vi "MyrioProject.vi"() -> ()   [LabVIEW 2018]
doc: "The myRIO Project template acquires acceleration data from the onboard accelerometer and displays the changes of acceleration values in a waveform chart."
uses:
  <vilib>/Platform/TimedLoop/XDataNode/timing_clust.ctl
  <vilib>/Platform/TimedLoop/XDataNode/nitl_modes.ctl
  <vilib>/Platform/TimedLoop/XDataNode/wakeup.ctl
  <vilib>/myRIO/Common/Instrument Driver Framework/myRIO v1.0/Encoder/typedefs/Encoder Signal Mode.ctl
  <vilib>/myRIO/Instrument Drivers/Onboard IO/PWM/typedefs/PWM Reference.ctl
  <vilib>/myRIO/Common/Instrument Driver Framework/Utilities/typedefs/myRIO Generic Hardware Reference.ctl
  <vilib>/myRIO/Common/Instrument Driver Framework/Utilities/typedefs/Hardware Version Enum.ctl
  <vilib>/myRIO/Common/Instrument Driver Framework/Utilities/typedefs/myRIO v1.0 Reference.ctl
  <vilib>/myRIO/Common/Instrument Driver Framework/Utilities/typedefs/Generic FPGA Reference.ctl
  <vilib>/myRIO/Common/Instrument Driver Framework/myRIO v1.0/PWM/typedefs/PWM Channels Enum.ctl
  <vilib>/myRIO/Instrument Drivers/Onboard IO/PWM/typedefs/PWM Configuration.ctl
  <vilib>/userdefined/High Color/nirio_resource_hc.ctl
  <vilib>/myRIO/Common/Instrument Driver Framework/myRIO v1.0/Encoder/typedefs/Encoder Configuration v1.0.ctl
  <vilib>/myRIO/Instrument Drivers/Onboard IO/Encoder/typedefs/Encoder Reference.ctl
  <vilib>/myRIO/Common/Instrument Driver Framework/myRIO v1.0/Encoder/typedefs/Encoder Channels Enum.ctl
  <vilib>/myRIO/Instrument Drivers/Onboard IO/DIO/typedefs/DIO Reference.ctl
  <vilib>/myRIO/Common/Instrument Driver Framework/myRIO v1.0/DIO/typedefs/DIO Channels List.ctl
  <vilib>/myRIO/Common/Instrument Driver Framework/myRIO v1.0/DIO/typedefs/DIO Channels Enum.ctl
  <vilib>/myRIO/Instrument Drivers/Onboard IO/AI/typedefs/AI Reference.ctl
  <vilib>/myRIO/Common/Instrument Driver Framework/myRIO v1.0/AI/typedefs/AI Channels List.ctl
  <vilib>/myRIO/Common/Instrument Driver Framework/myRIO v1.0/AI/typedefs/AI Channels Enum.ctl
  <vilib>/myRIO/Common/Instrument Driver Framework/Utilities/typedefs/Analog Scaling Constants List.ctl
  <vilib>/myRIO/Common/Instrument Driver Framework/Utilities/typedefs/Analog Scaling Constants.ctl
  <vilib>/myRIO/Common/Instrument Driver Framework/myRIO v1.0/PWM/vis/myRIO v1.1 Open PWM.vi
  <vilib>/myRIO/Common/Instrument Driver Framework/myRIO v1.0/Encoder/vis/myRIO v1.1 Open Encoder.vi
  <vilib>/myRIO/Common/Instrument Driver Framework/Utilities/vis/Is FPGA Ref Available.vi
  <vilib>/myRIO/Common/Instrument Driver Framework/myRIO v1.0/AI/vis/myRIO v1.1 Open AI.vi
  <vilib>/myRIO/Common/Instrument Driver Framework/myRIO v1.0/DIO/vis/myRIO v1.1 Open DIO.vi
  <vilib>/myRIO/Instrument Drivers/Onboard IO/PWM/vis/Set Duty Cycle and Frequency.vi
  <vilib>/myRIO/Instrument Drivers/Onboard IO/DIO/vis/Write.vi
  <vilib>/myRIO/Common/Instrument Driver Framework/Utilities/vis/Validate Channels.vi
  <vilib>/myRIO/Common/Instrument Driver Framework/myRIO v1.0/PWM/vis/myRIO v1.0 Reserve PWM.vi
  <vilib>/myRIO/Common/Instrument Driver Framework/myRIO v1.0/Encoder/vis/myRIO v1.0 Reserve Encoder.vi
  <vilib>/myRIO/Common/Instrument Driver Framework/myRIO v1.0/AI/vis/myRIO v1.0 Reserve AI.vi
  <vilib>/myRIO/Common/Instrument Driver Framework/myRIO v1.0/DIO/vis/myRIO v1.0 Reserve DIO.vi
  <vilib>/myRIO/Common/Instrument Driver Framework/myRIO v1.0/Encoder/vis/myRIO v1.0 Close Encoder.vi
  <vilib>/myRIO/Common/Instrument Driver Framework/myRIO v1.0/PWM/vis/myRIO v1.0 Close PWM.vi
  <vilib>/myRIO/Common/Instrument Driver Framework/myRIO v1.0/PWM/vis/myRIO v1.0 Build MUX Configuration PWM.vi
  <vilib>/myRIO/Common/Instrument Driver Framework/myRIO v1.0/Resource Manager/vis/myRIO v1.0 Reserve Channel List.vi
  <vilib>/myRIO/Common/Instrument Driver Framework/myRIO v1.0/Encoder/vis/myRIO v1.0 Build MUX Configuration Encoder.vi
  <vilib>/myRIO/Common/Instrument Driver Framework/myRIO v1.0/AI/vis/myRIO v1.0 Build MUX Configuration AI.vi
  <vilib>/myRIO/Common/Instrument Driver Framework/myRIO v1.0/DIO/vis/myRIO v1.0 Build MUX Configuration DIO.vi
  <vilib>/myRIO/Common/Instrument Driver Framework/myRIO v1.0/Encoder/vis/myRIO v1.0 Unreserve Encoder.vi
  <vilib>/myRIO/Common/Instrument Driver Framework/myRIO v1.0/PWM/vis/myRIO v1.0 Unreserve PWM.vi
  <vilib>/myRIO/Common/Instrument Driver Framework/myRIO v1.0/Resource Manager/vis/myRIO v1.0 Create Configuration List.vi
  <vilib>/myRIO/Common/Instrument Driver Framework/myRIO v1.0/Resource Manager/vis/myRIO v1.0 Reserve Channel.vi
  <vilib>/myRIO/Common/Instrument Driver Framework/myRIO v1.0/Resource Manager/vis/myRIO v1.0 Unreserve Channel.vi
  <vilib>/myRIO/Common/Instrument Driver Framework/myRIO v1.0/Resource Manager/vis/myRIO v1.0 Unreserve Channel List.vi
  <vilib>/myRIO/Common/Instrument Driver Framework/myRIO v1.0/Resource Manager/vis/myRIO v1.0 Build Mutex Name.vi
  <vilib>/Utility/VariantDataType/GetNumericInfo.vi
  <vilib>/Utility/error.llb/Error Cluster From Error Code.vi
  <vilib>/myRIO/Common/Instrument Driver Framework/myRIO v1.0/myRIO v1.1 Open.vi
  <vilib>/myRIO/Common/Instrument Driver Framework/Utilities/vis/IO Manager.vi
  <vilib>/myRIO/Common/Instrument Driver Framework/Utilities/vis/Configuration Manager.vi
  <vilib>/myRIO/Common/Instrument Driver Framework/myRIO v1.0/Resource Manager/vis/myRIO v1.0 Configure IO.vi
  <vilib>/myRIO/Common/Instrument Driver Framework/myRIO v1.0/myRIO v1.0 Close.vi
  <vilib>/myRIO/Common/Instrument Driver Framework/myRIO v1.0/PWM/vis/myRIO v1.0 Write PWM.vi
  <vilib>/myRIO/Common/Instrument Driver Framework/myRIO v1.0/Encoder/vis/myRIO v1.0 Configure Encoder.vi
  <vilib>/myRIO/Common/Instrument Driver Framework/myRIO v1.0/Encoder/vis/myRIO v1.0 Enable Encoder.vi
  <vilib>/myRIO/Common/Instrument Driver Framework/myRIO v1.0/DIO/vis/myRIO v1.0 Read DIO.vi
  <vilib>/myRIO/Common/Instrument Driver Framework/myRIO v1.0/AI/vis/myRIO v1.0 Get Scaling Constants AI.vi
  <vilib>/myRIO/Common/Instrument Driver Framework/myRIO v1.0/AI/vis/myRIO v1.0 Read AI.vi
  <vilib>/myRIO/Common/Instrument Driver Framework/myRIO v1.0/Encoder/vis/myRIO v1.0 Read Encoder.vi
  <vilib>/myRIO/Common/Instrument Driver Framework/myRIO v1.0/DIO/vis/myRIO v1.0 Write DIO.vi
  <vilib>/myRIO/Common/Instrument Driver Framework/myRIO v1.0/Encoder/vis/myRIO v1.0 Shutdown Encoder.vi
  <vilib>/myRIO/Common/Instrument Driver Framework/myRIO v1.0/PWM/vis/myRIO v1.0 Shutdown PWM.vi
  <vilib>/platform/TimedLoop/XDataNode/XDataNode.xnode
  <vilib>/myRIO/Instrument Drivers/Onboard IO/PWM/vis/myRIO PWM Open.xnode
  <vilib>/myRIO/Instrument Drivers/Onboard IO/Encoder/vis/myRIO Encoder Open.xnode
  <vilib>/myRIO/Express VI/Onboard IO/PWM/PWM Express VI.xnode
  <vilib>/myRIO/Express VI/Onboard Devices/Button/Button Express VI.xnode
  <vilib>/myRIO/Instrument Drivers/Onboard IO/DIO/vis/myRIO DIO Open.xnode
  <vilib>/myRIO/Express VI/Onboard IO/AI/AI Express VI.xnode
  <vilib>/myRIO/Instrument Drivers/Onboard IO/AI/vis/myRIO AI Open.xnode
  <vilib>/myRIO/Express VI/Onboard IO/DO/DO Express VI.xnode
  <vilib>/Platform/TimedLoop/XDataNode/XDNodeRunTimeDep.lvlib
  <vilib>/myRIO/Instrument Drivers/Onboard IO/Encoder/Encoder.lvlib
  <vilib>/myRIO/Instrument Drivers/Onboard IO/PWM/PWM.lvlib
  <vilib>/myRIO/Instrument Drivers/Onboard IO/DIO/DIO.lvlib
  <vilib>/myRIO/Instrument Drivers/Onboard IO/AI/AI.lvlib
panel:
  in  "MANUAL 2":bool
  in  "Stop Button":bool
  in  "Start":bool
  out "element":dbl
  out "element 2":dbl
  out "subarray 2":dbl[][](array[numeric])
  out "subarray":dbl[][](array[numeric])
  out "vectores":dbl[][][](array[numeric])
  in  "saturacion":dbl
  in  "Duty Cycle 2":dbl(slide)=0.5 scale=0.05..0.1
  in  "Duty Cycle":dbl(slide)=0.5 scale=0.05..0.1
  in  "Reset Counter 2":bool
  in  "Reset Counter":bool
  out "stallRojo (A/AI3 (Pin 9))":dbl
  out "stallBlanco (A/AI2 (Pin 7))":dbl
  out "sensor2 (A/AI1 (Pin 5))":dbl
  out "A/AI0 (Pin 3)":dbl
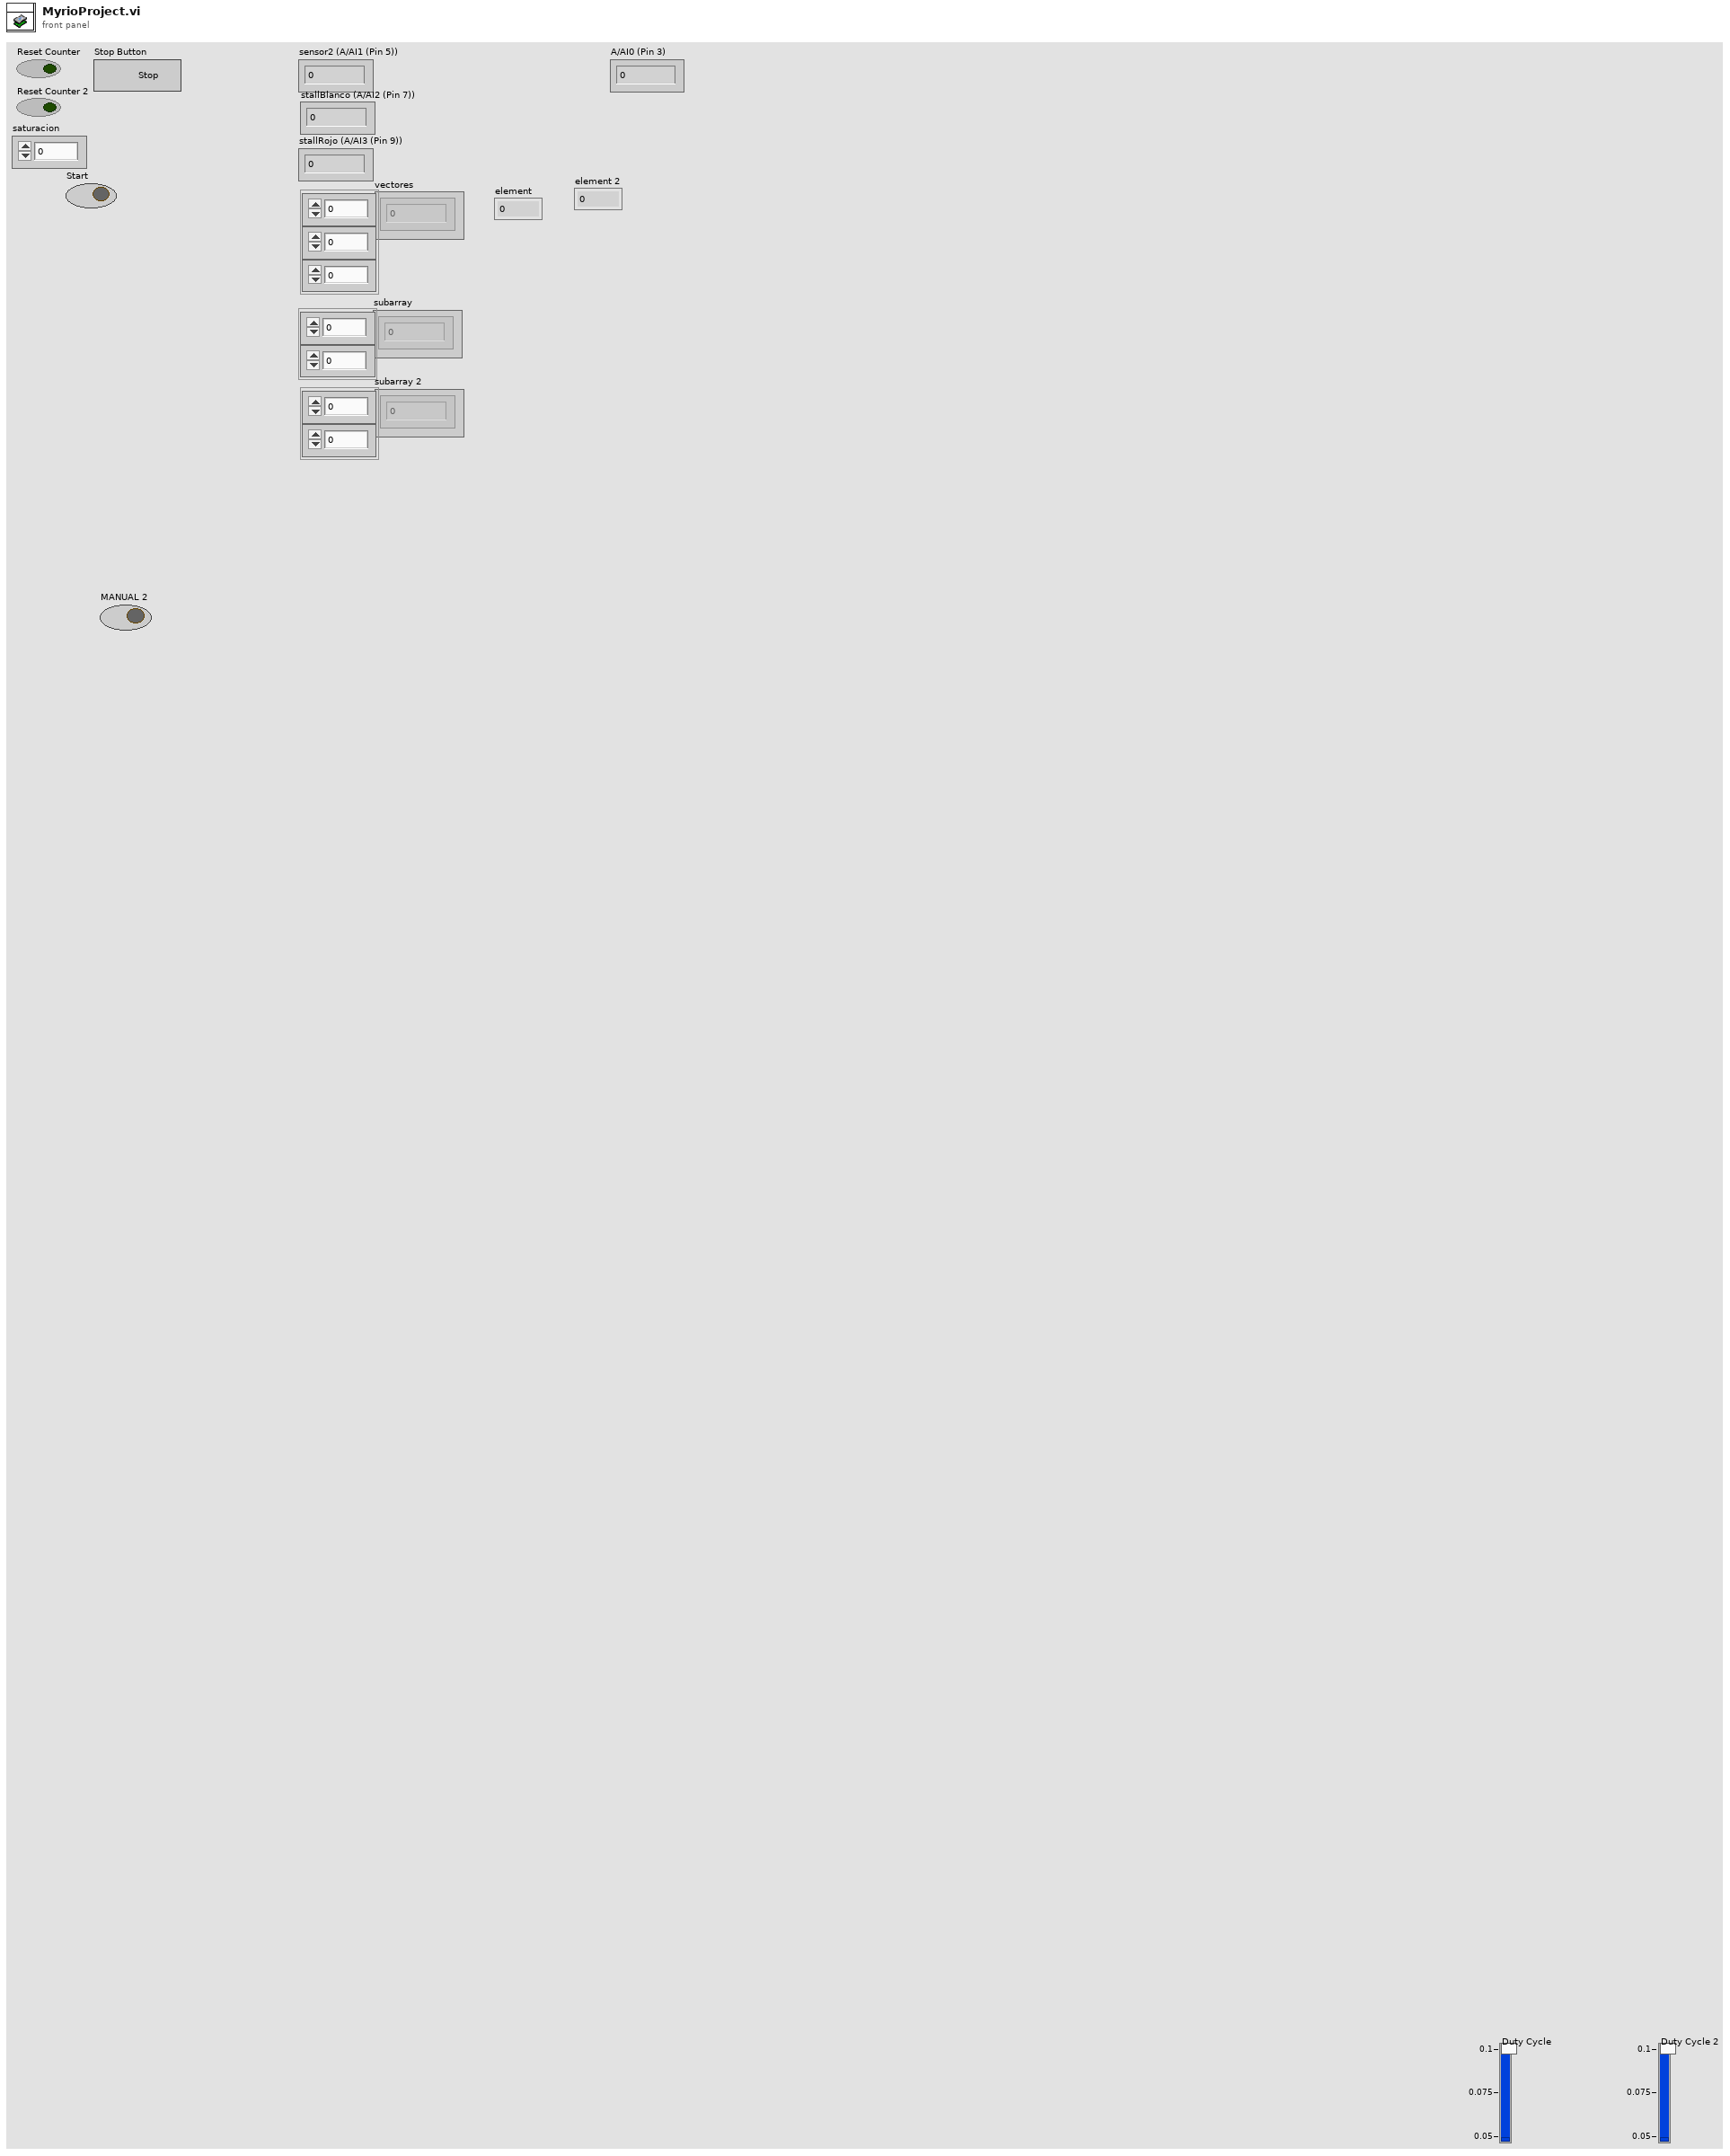
[diagram p1: front panel]
types:
  T1 = typedef "Encoder Signal Mode.ctl" = enum16{"Quadrature phase signal", "Step and direction signal"}
  T2 = typedef "PWM.lvlib/PWM Reference.ctl" = cluster{"myRIO Reference":T3, "PWM Channels Enum":T7, "PWM Configuration":T8}
  T3 = typedef "myRIO Generic Hardware Reference.ctl" = cluster{"myRIO Model":T4, "myRIO Hardware Reference":T5}
  T4 = typedef "Hardware Version Enum.ctl" = enum16{"Unknown", "myRIO-1900", "myRIO-1950", "roboRIO", "NI ELVIS RIO CM", "ELVIS III"}
  T5 = typedef "myRIO v1.0 Reference.ctl" = cluster{"Generic FPGA Reference":T6, "Allow multiple opens":bool}
  T6 = typedef "Generic FPGA Reference.ctl" = refnum<k20>
  T7 = typedef "PWM Channels Enum.ctl" = enum16{"Not Connected", "C/PWM0", "C/PWM1", "A/PWM0", "A/PWM1", "A/PWM2", "A/PWM3", "A/PWM4", "A/PWM5", "A/PWM6", "A/PWM7", "A/PWM8", "A/PWM9", "A/PWM10", "A/PWM11", "A/PWM12", "A/PWM13", "A/PWM14", "A/PWM15", "A/PWM16", "A/PWM17", "A/PWM18", "A/PWM19", "B/PWM0", "B/PWM1", "B/PWM2", "B/PWM3", "B/PWM4", "B/PWM5", "B/PWM6", "B/PWM7", "B/PWM8", "B/PWM9", "B/PWM10", "B/PWM11", "B/PWM12", "B/PWM13", "B/PWM14", "B/PWM15", "B/PWM16", "B/PWM17", "B/PWM18", "B/PWM19", "PWM/PWM0", "PWM/PWM1", "PWM/PWM2", "PWM/PWM3", "PWM/PWM4", "PWM/PWM5", "PWM/PWM6", "PWM/PWM7", "PWM/PWM8", "PWM/PWM9"}
  T8 = typedef "PWM.lvlib/PWM Configuration.ctl" = cluster{"Frequency":dbl, "Duty Cycle":dbl}
  T9 = typedef "Encoder.lvlib/Encoder Reference.ctl" = cluster{"myRIO Reference":T3, "Encoder Channels Enum":T10}
  T10 = typedef "Encoder Channels Enum.ctl" = enum16{"Not Connected", "C/ENC0", "C/ENC1", "A/ENC", "A/ENC0", "A/ENC1", "A/ENC2", "A/ENC3", "A/ENC4", "A/ENC5", "A/ENC6", "A/ENC7", "A/ENC8", "A/ENC9", "B/ENC", "B/ENC0", "B/ENC1", "B/ENC2", "B/ENC3", "B/ENC4", "B/ENC5", "B/ENC6", "B/ENC7", "B/ENC8", "B/ENC9", "DIO/ENC0", "DIO/ENC1", "DIO/ENC2", "DIO/ENC3", "DIO/ENC4"}
  T11 = typedef "XDNodeRunTimeDep.lvlib/timing_clust.ctl" = cluster{"Expected End [f-1]":u64, "Actual End [f-1]":u64, "Finished Late? [f-1]":bool, "Expected End [i-1]":u64, "Actual End [i-1]":u64, "Finished Late? [i-1]":bool, "Expected Start [i]":u64, "Actual Start [i]":u64, "Expected Start [f]":u64, "Actual Start [f]":u64, "Source Name":string, "Structure Name":string, "Period":i64, "Deadline":i64, "Offset":i64, "Start":i64, "Priority":i32, "Timeout":i32, "Mode":T12, "Wakeup Reason":T13, "Error":errorcluster, "Source Type":string, "Secondary Source Type":string, "Global End Time":u64, "Global Start Time":u64, "Frame Duration":u64, "Iteration Duration":u64, "Assigned CPU":i32, "I/O Scan Engine Mode":u32}
  T12 = typedef "XDNodeRunTimeDep.lvlib/nitl_modes.ctl" = enum32{"No Change", "Process missed periods, maintain original phase", "Discard missed periods, maintain original phase", "Process missed periods, ignore original phase", "Discard missed periods, ignore original phase"}
  T13 = typedef "XDNodeRunTimeDep.lvlib/wakeup.ctl" = enum32{"Normal", "Aborted", "Asynchronous wakeup", "Timing source error", "Timed loop error", "Timeout"}
  T14 = enum16{"normal", "grande-Sensor", "grande home", "peque-sensor", "peque- home", "peque-reset"}
  T15 = typedef "nirio_resource_hc.ctl" = tag
  T16 = enum16{"normal", "grande-Sensor", "grande home", "peque-sensor", "peque- home"}
  T17 = typedef "AI.lvlib/AI Reference.ctl" = cluster{"myRIO Reference":T3, "AI Channels List":T18, "AI Scaling Constants List":T20}
  T18 = typedef "AI Channels List.ctl" = T19[]
  T19 = typedef "AI Channels Enum.ctl" = enum16{"Not Connected", "AudioIn/Left", "AudioIn/Right", "C/AI0", "C/AI1", "A/AI0", "A/AI1", "A/AI2", "A/AI3", "A/AI4", "A/AI5", "A/AI6", "A/AI7", "B/AI0", "B/AI1", "B/AI2", "B/AI3", "B/AI4", "B/AI5", "B/AI6", "B/AI7", "AI/AI0", "AI/AI1", "AI/AI2", "AI/AI3", "A/AI0 (DIFF)", "A/AI1 (DIFF)", "A/AI2 (DIFF)", "A/AI3 (DIFF)", "B/AI0 (DIFF)", "B/AI1 (DIFF)", "B/AI2 (DIFF)", "B/AI3 (DIFF)"}
  T20 = typedef "Analog Scaling Constants List.ctl" = T21[]
  T21 = typedef "Analog Scaling Constants.ctl" = cluster{"LSB Weight (Volts)":dbl, "Offset (Volts)":dbl, "Signed?":bool}
  T22 = typedef "DIO.lvlib/DIO Reference.ctl" = cluster{"myRIO Reference":T3, "DIO Channels List":T23}
  T23 = typedef "DIO Channels List.ctl" = T24[]
  T24 = typedef "DIO Channels Enum.ctl" = enum16{"Not Connected", "C/DIO0", "C/DIO1", "C/DIO2", "C/DIO3", "C/DIO4", "C/DIO5", "C/DIO6", "C/DIO7", "A/DIO0", "A/DIO1", "A/DIO2", "A/DIO3", "A/DIO4", "A/DIO5", "A/DIO6", "A/DIO7", "A/DIO8", "A/DIO9", "A/DIO10", "A/DIO11", "A/DIO12", "A/DIO13", "A/DIO14", "A/DIO15", "A/DIO16", "A/DIO17", "A/DIO18", "A/DIO19", "B/DIO0", "B/DIO1", "B/DIO2", "B/DIO3", "B/DIO4", "B/DIO5", "B/DIO6", "B/DIO7", "B/DIO8", "B/DIO9", "B/DIO10", "B/DIO11", "B/DIO12", "B/DIO13", "B/DIO14", "B/DIO15", "B/DIO16", "B/DIO17", "B/DIO18", "B/DIO19", "LED0", "LED1", "LED2", "LED3", "Button0", "DIO/DIO0", "DIO/DIO1", "DIO/DIO2", "DIO/DIO3", "DIO/DIO4", "DIO/DIO5", "DIO/DIO6", "DIO/DIO7", "DIO/DIO8", "DIO/DIO9", "SPI/CS0", "SPI/CS1", "SPI/CS2", "SPI/CS3", "LED RADIO (Green)", "LED RADIO (Red)", "LED COMM (Green)", "LED COMM (Red)", "LED MODE (Green)", "LED MODE (Red)"}
  T25 = cluster{"Double":dbl, dbl, "Counter Value":i32, "seconds since 1Jan1904":timestamp, "Double":dbl, dbl, dbl}
  T26 = cluster{"Double":dbl, "dbl Scaled Value":dbl, "Output":dbl, "seconds since 1Jan1904":timestamp, dbl, dbl, dbl}
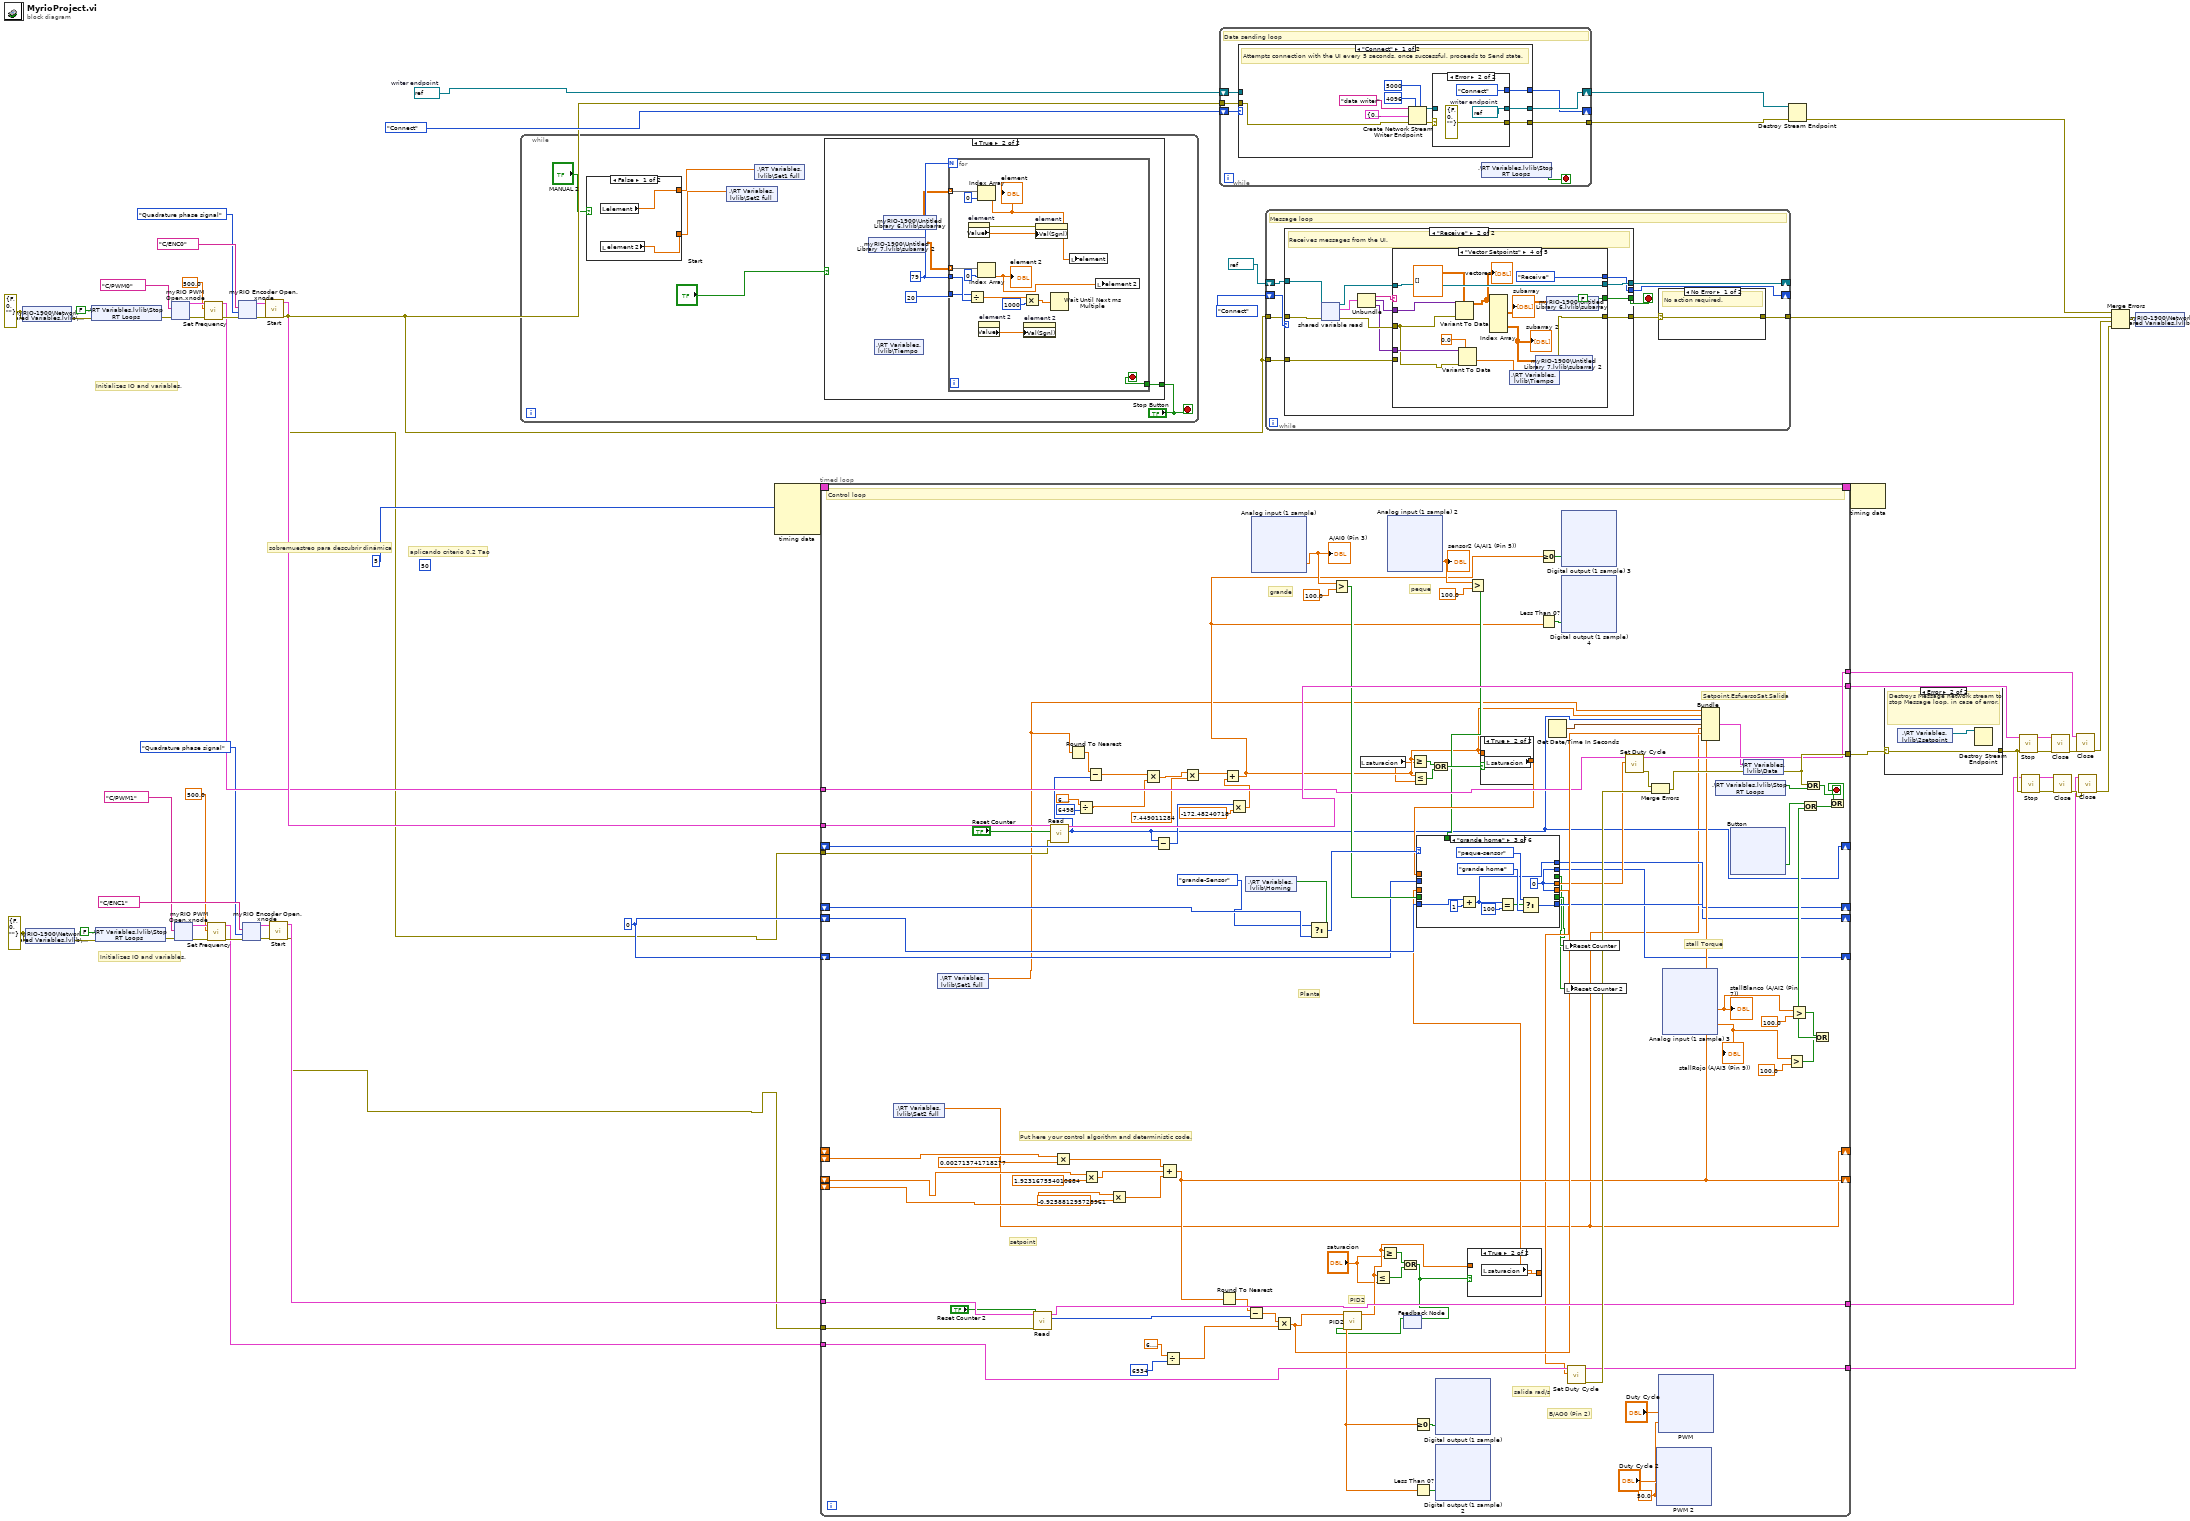
[diagram p0: block diagram]
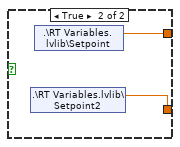
[diagram p2: hidden frame]
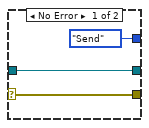
[diagram p5: hidden frame]
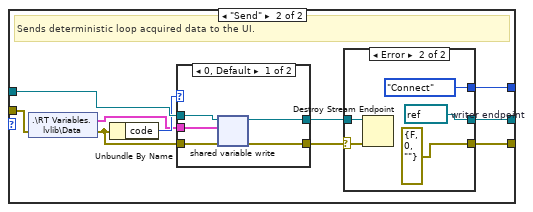
[diagram p6: hidden frame]
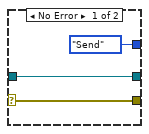
[diagram p7: hidden frame]
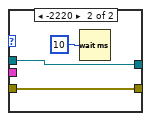
[diagram p8: hidden frame]
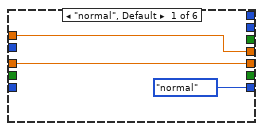
[diagram p9: hidden frame]
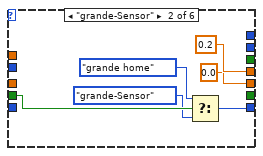
[diagram p10: hidden frame]
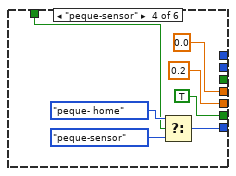
[diagram p11: hidden frame]
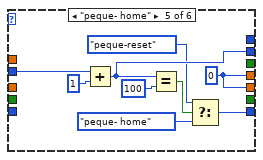
[diagram p12: hidden frame]
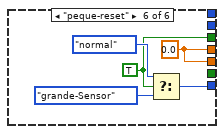
[diagram p13: hidden frame]
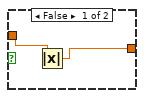
[diagram p14: hidden frame]
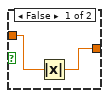
[diagram p15: hidden frame]
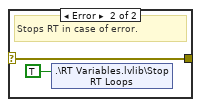
[diagram p16: hidden frame]
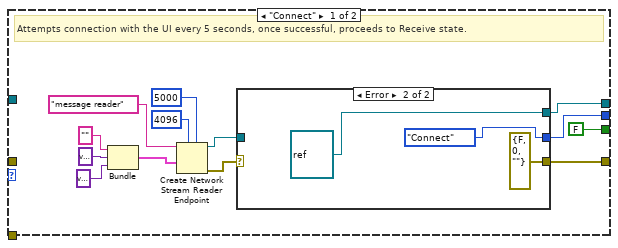
[diagram p17: hidden frame]
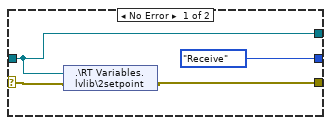
[diagram p18: hidden frame]
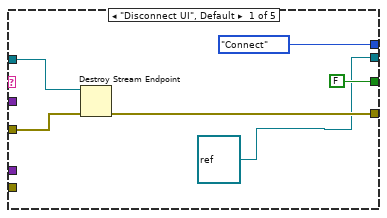
[diagram p19: hidden frame]
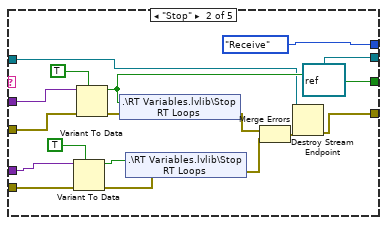
[diagram p20: hidden frame]
diagram:
  w3 = 0
  (unwired) 50
  w13 = refnum<k21> refnum  # writer endpoint
  w26 = errorcluster {"status"=FALSE, "code"=0, "source"=""} ("error IO")
  w48 = errorcluster {"status"=FALSE, "code"=0, "source"=""} ("error IO")
  # "aplicando criterio 0.2 Tao"
  # "sobremuestreo para descubrir dinámica"
  # "Initializes IO and variables."
  # "Initializes IO and variables."
  n1 = shared-variable "myRIO-1900\\Network Shared Variables.lvlib\\error IO"(w48, error in=w48) -> (error out=w49:errorcluster)
  n2 = shared-variable "myRIO-1900\\Network Shared Variables.lvlib\\error IO"(w26, error in=w26) -> (error out=w27:errorcluster)
  n3 = shared-variable ".\\RT Variables.lvlib\\Stop RT Loops"(FALSE ("Stop RT Loops"), error in=w49) -> (error out=w36:errorcluster)
  n4 = shared-variable ".\\RT Variables.lvlib\\Stop RT Loops"(FALSE ("Stop RT Loops"), error in=w27) -> (error out=w19:errorcluster)
  n5 = xnode "myRIO PWM Open.xnode"("error in (no error)"=w36, "Channel Name"=tag "C/PWM0") -> ("error out"=w38:errorcluster, "PWM Ref Out"=w37:T2)  [unwired: 1 in]
  n6 = xnode "myRIO PWM Open.xnode"("error in (no error)"=w19, "Channel Name"=tag "C/PWM1") -> ("error out"=w21:errorcluster, "PWM Ref Out"=w20:T2)  [unwired: 1 in]
  n7 = call <vilib>:"Set Frequency.vi"("error in (no error)"=w38, "Frequency [Hz]"=500.0, "PWM Ref In"=w37) -> ("error out"=w35:errorcluster, "PWM Ref Out"=w32:T2)  [unwired: 6 in]
  n8 = call <vilib>:"Set Frequency.vi"("error in (no error)"=w21, "Frequency [Hz]"=500.0, "PWM Ref In"=w20) -> ("error out"=w18:errorcluster, "PWM Ref Out"=w14:T2)  [unwired: 6 in]
  n9 = xnode "myRIO Encoder Open.xnode"("error in (no error)"=w35, "Channel Name"=tag "C/ENC0", "Encoder Signal Mode"=Encoder_Signal_Mode."Quadrature phase signal") -> ("error out"=w45:errorcluster, "Encoder Ref Out"=w44:T9)  [unwired: 2 in]
  n10 = xnode "myRIO Encoder Open.xnode"("error in (no error)"=w18, "Channel Name"=tag "C/ENC1", "Encoder Signal Mode"=Encoder_Signal_Mode."Quadrature phase signal") -> ("error out"=w24:errorcluster, "Encoder Ref Out"=w23:T9)  [unwired: 2 in]
  n11 = call <vilib>:"Start.vi"("error in (no error)"=w45, "Encoder Ref In"=w44) -> ("error out"=w2:errorcluster, "Encoder Ref Out"=w42:T9)  [unwired: 8 in]
  n12 = call <vilib>:"Start.vi"("error in (no error)"=w24, "Encoder Ref In"=w23) -> ("error out"=w1:errorcluster, "Encoder Ref Out"=w15:T9)  [unwired: 8 in]
  n13 = while {
    stop <- "Stop Button" stop-if-true
    n14 = case shown="False" "MANUAL 2" {
      tunnel: [w66 w68] -> w62
      tunnel: [w65 w67] -> w61
      frame False {
        n15 = local read "element"() -> (w65:dbl)
        n16 = local read "element 2"() -> (w66:dbl)
      }
      frame True {
        n17 = shared-variable ".\\RT Variables.lvlib\\Setpoint2"() -> (w68:dbl)  [unwired: 1 in, 1 out]
        n18 = shared-variable ".\\RT Variables.lvlib\\Setpoint"() -> (w67:dbl)  [unwired: 1 in, 1 out]
      }
    }
    n19 = shared-variable ".\\RT Variables.lvlib\\Set2 full"(w62) -> ()  [unwired: 1 in, 1 out]
    n20 = shared-variable ".\\RT Variables.lvlib\\Set1 full"(w61) -> ()  [unwired: 1 in, 1 out]
    n21 = case shown="True" "Start" {
      tunnel: "Stop Button" -> [_ w70]
      frame False {
      }
      frame True {
        w73 = 79
        n22 = shared-variable "myRIO-1900\\Untitled Library 7.lvlib\\subarray 2"() -> (w71:dbl[][])  [unwired: 1 in, 1 out]
        n23 = shared-variable ".\\RT Variables.lvlib\\Tiempo"() -> ()  [unwired: 1 in, 2 out]
        n24 = shared-variable "myRIO-1900\\Untitled Library 6.lvlib\\subarray"() -> (w72:dbl[][])  [unwired: 1 in, 1 out]
        n25 = for {
          N: w73 -> [_]
          tunnel: w73 -> [w86]
          tunnel: w72 -> [w85] mode=indexing
          tunnel: 20 -> [w83]
          tunnel: w71 -> [w81] mode=indexing
          tunnel: w70 -> [w74]
          stop <- w74 stop-if-true
          n26 = property on="element" class="DigNum (strict)"() -> (error out=w79:errorcluster, "Value"=w80:dbl)  [unwired: 2 in, 1 out]
          n27 = Divide(x=w83, y=w86) -> (x/y=w88:dbl)
          n28 = Index Array(array=w85, index=0) -> (element=w78:dbl)
          "element" <- w78
          n29 = Index Array(array=w81, index=0) -> (element=w75:dbl)
          "element 2" <- w75
          n30 = property on="element 2" class="DigNum (strict)"() -> ("Value"=w77:dbl)  [unwired: 2 in, 2 out]
          n31 = Multiply(x=w88, y=1000) -> (x*y=w76:dbl)
          n32 = property on="element 2" class="DigNum (strict)"("Val(Sgnl)"=w77) -> ()  [unwired: 2 in, 2 out]
          n33 = property on="element" class="DigNum (strict)"(error in=w79, "Val(Sgnl)"=w80) -> ()  [unwired: 1 in, 2 out]
          n34 = Wait Until Next ms Multiple(millisecond multiple=w76) -> ()  [unwired: 1 out]
          n35 = local write "element"(w78) -> ()
          n36 = local write "element 2"(w75) -> ()
        }
      }
    }
  }
  n37 = node-c288(i64 5 ("Period")) -> (w59:T11)  [unwired: 3 in]
  n38 = timed-loop {
    timing: w59 -> [_]
    timing-out: [_] -> w58
    tunnel: [w187] -> w47
    tunnel: w42 -> [w147]
    tunnel: [w146] -> w39
    tunnel: w32 -> [w127]
    tunnel: [w186] -> w31
    tunnel: w15 -> [w183]
    tunnel: w14 -> [w182]
    tunnel: [w178] -> w8
    tunnel: [w177] -> w7
    shift-right: [w89] -> _
    shift-left: _ -> [_]
    shift-left: _ -> [w162]
    shift-right: [w151] -> _
    shift-left: _ -> [w161]
    shift-left: _ -> [w160]
    shift-right: [w124] -> _
    shift-left: _ -> [w123]
    shift-right: [w121] -> _
    shift-left: w3 -> [w120]
    shift-right: [w116] -> _
    shift-left: w3 -> [w115]
    shift-right: [w100] -> _
    shift-left: _ -> [w101]
    tunnel: w1 -> [w92]
    tunnel: w2 -> [w91]
    stop <- w175 stop-if-true
    w96 = 50.0 ("Frequency [Hz]")
    # "peque"
    # "grande"
    # "stall Torque"
    # "Setpoint,EsfuersoSat,Salida"
    # "setpoint"
    # "PID2"
    # "Put here your control algorithm and deterministic code."
    # "Planta"
    # "salida rad/s"
    # "B/AO0 (Pin 2)"
    # "Control loop"
    n39 = shared-variable ".\\RT Variables.lvlib\\Set2 full"() -> (w89:dbl)  [unwired: 1 in, 1 out]
    n40 = shared-variable ".\\RT Variables.lvlib\\Set1 full"() -> (w90:dbl)  [unwired: 1 in, 1 out]
    n41 = call <vilib>:"Read.vi"("error in (no error)"=w92, "Reset Counter"="Reset Counter 2", "Encoder Ref In"=w183) -> ("Counter Value"=w155:i32, "Encoder Ref Out"=w178:T9)  [unwired: 4 in, 3 out]
    n42 = call <vilib>:"Read.vi"("error in (no error)"=w91, "Reset Counter"="Reset Counter", "Encoder Ref In"=w147) -> ("Counter Value"=w100:i32, "Encoder Ref Out"=w146:T9)  [unwired: 4 in, 3 out]
    n43 = Multiply(x=w162, y=0.002713741718277) -> (x*y=w164:dbl)
    n44 = Round To Nearest(number=w90) -> (nearest integer value=w145:dbl)
    n45 = Divide(x=6.283185307179586, y=6498) -> (x/y=w103:dbl)
    n46 = Multiply(x=w161, y=1.923167554010684) -> (x*y=w165:dbl)
    n47 = Subtract(x=w145, y=w100) -> (x-y=w102:dbl)
    n48 = Multiply(x=w160, y=-0.925881295728961) -> (x*y=w163:dbl)
    n49 = Multiply(x=w102, y=w103) -> (x*y=w109:dbl)
    n50 = Subtract(x=w100, y=w101) -> (x-y=w104:i32)
    n51 = Compound Arithmetic op=ADD(w164, w165, w163) -> (w151:dbl)
    n52 = Divide(x=6.283185307179586, y=6534) -> (x/y=w153:dbl)
    n53 = Multiply(x=w109, y=7.449011284) -> (x*y=w107:dbl)
    n54 = Round To Nearest(number=w151) -> (nearest integer value=w150:dbl)
    n55 = Multiply(x=w104, y=-172.48240718) -> (x*y=w105:dbl)
    n56 = Add(x=w107, y=w105) -> (x+y=w99:dbl)
    n57 = shared-variable ".\\RT Variables.lvlib\\Homing"() -> (w128:bool)  [unwired: 1 in, 1 out]
    n58 = Subtract(x=w150, y=w155) -> (x-y=w154:dbl)
    n59 = xnode "Analog input (1 sample)"() -> ("A/AI0 (Pin 3)"=w141:dbl)  [unwired: 1 in, 1 out]
    "A/AI0 (Pin 3)" <- w141
    n60 = Multiply(x=w154, y=w153) -> (x*y=w152:dbl)
    n61 = Select(t=T14."grande-Sensor" ("Enum"), s=w128, f=w123) -> (s? t:f=w129:T14)
    n62 = Greater?(x=w141, y=100.0) -> (0:w122:bool)
    n63 = local read "saturacion"() -> (w94:dbl)
    n64 = xnode "Analog input (1 sample) 2"() -> ("sensor2 (A/AI1 (Pin 5))"=w138:dbl)  [unwired: 1 in, 1 out]
    "sensor2 (A/AI1 (Pin 5))" <- w138
    n65 = feedback #1() -> (w158:bool)  [unwired: 1 in]
    n66 = call "PID2.vi"("Boolean"=w158, "Numeric in"=w152) -> ("Numeric out"=w159:dbl)  [unwired: 9 in]
    n67 = Less Or Equal?(x=w159, y="saturacion") -> (x <= y?=w171:bool)
    n68 = Greater Or Equal?(x=w159, y="saturacion") -> (x >= y?=w172:bool)
    n69 = Or(x=w172, y=w171) -> (x .or. y?=w157:bool)
    n70 = feedback-in #1(w157) -> ()
    n71 = Greater Or Equal?(x=w99, y=w94) -> (x >= y?=w174:bool)
    n72 = Less Or Equal?(x=w99, y=w94) -> (x <= y?=w173:bool)
    n73 = Greater Or Equal To 0?(x=w159) -> (x >= 0?=w170:bool)
    n74 = Less Than 0?(x=w159) -> (x < 0?=w169:bool)
    n75 = Or(x=w174, y=w173) -> (x .or. y?=w144:bool)
    n76 = xnode "Digital output (1 sample)"("A/DIO0 (Pin 11)"=w170) -> ()  [unwired: 1 in, 1 out]
    n77 = xnode "Digital output (1 sample) 2"("A/DIO1 (Pin 13)"=w169) -> ()  [unwired: 1 in, 1 out]
    n78 = case shown="True" w157 {
      tunnel: [w551 w553] -> w119
      tunnel: w159 -> [w552 _]
      frame False {
        n79 = Absolute Value(x=w552) -> (abs(x)=w551:dbl)
      }
      frame True {
        n80 = local read "saturacion"() -> (w553:dbl)
      }
    }
    n81 = Greater?(x=w138, y=100.0) -> (0:w117:bool)
    n82 = case shown="True" w144 {
      tunnel: [w554 w556] -> w126
      tunnel: w99 -> [w555 _]
      frame False {
        n83 = Absolute Value(x=w555) -> (abs(x)=w554:dbl)
      }
      frame True {
        n84 = local read "saturacion"() -> (w556:dbl)
      }
    }
    n85 = case shown="\"grande home\"" w129 {
      tunnel: w126 -> [w262 _ _ _ _ _]
      tunnel: [w262 0.2 ("f") w269 0.0 ("f") w289 w297] -> w125
      tunnel: [T16."normal" ("Enum") w264 w270 w280 w288 w295] -> w124
      tunnel: w122 -> [_ w267 _ _ _ _]
      tunnel: [_ _ w273 _ _ _] -> w121
      tunnel: w120 -> [_ _ w274 _ _ _]
      tunnel: w119 -> [w260 _ _ _ _ _]
      tunnel: [w260 0.0 ("f") w269 0.2 ("f") w289 w297] -> w118
      tunnel: w117 -> [_ _ _ w281 _ _]
      tunnel: [_ _ w269 _ w287 _] -> w116
      tunnel: w115 -> [_ _ _ _ w286 _]
      tunnel: [_ _ _ TRUE _ _] -> w112
      tunnel: [_ _ _ _ _ w294] -> w110
      frame "normal", Default {
      }
      frame "grande-Sensor" {
        n86 = Select(t=T16."grande home" ("Enum"), s=w267, f=T16."grande-Sensor" ("Enum")) -> (s? t:f=w264:T16)
      }
      frame "grande home" {
        w269 = 0
        n87 = Add(x=w274, y=1) -> (x+y=w273:i32)
        n88 = Equal?(x=w273, y=100) -> (x = y?=w271:bool)
        n89 = Select(t=T16."peque-sensor" ("Enum"), s=w271, f=T16."grande home" ("Enum")) -> (s? t:f=w270:T16)
      }
      frame "peque-sensor" {
        n90 = Select(t=T16."peque- home" ("Enum"), s=w281, f=T16."peque-sensor" ("Enum")) -> (s? t:f=w280:T16)
      }
      frame "peque- home" {
        w289 = 0
        n91 = Add(x=w286, y=1) -> (x+y=w287:i32)
        n92 = Equal?(x=w287, y=100) -> (x = y?=w293:bool)
        n93 = Select(t=T14."peque-reset" ("Enum"), s=w293, f=T16."peque- home" ("Enum")) -> (s? t:f=w288:T14)
      }
      frame "peque-reset" {
        w294 = TRUE
        w297 = 0.0 ("f")
        n94 = Select(t=T16."normal" ("Enum"), s=w294, f=T14."grande-Sensor" ("Enum")) -> (s? t:f=w295:T14)
      }
    }
    n95 = Greater Or Equal To 0?(x=w99) -> (x >= 0?=w142:bool)
    n96 = Less Than 0?(x=w99) -> (x < 0?=w143:bool)
    n97 = Get Date/Time In Seconds() -> (seconds since 1Jan1904=w189:timestamp)
    n98 = xnode "Digital output (1 sample) 3"("A/DIO2 (Pin 15)"=w142) -> ()  [unwired: 1 in, 1 out]
    n99 = xnode "Digital output (1 sample) 4"("A/DIO3 (Pin 17)"=w143) -> ()  [unwired: 1 in, 1 out]
    n100 = local write "Reset Counter"(w112) -> ()
    n101 = local write "Reset Counter 2"(w110) -> ()
    n102 = call <vilib>:"Set Duty Cycle.vi"("Duty Cycle"=w118, "PWM Ref In"=w182) -> ("error out"=w181:errorcluster, "PWM Ref Out"=w177:T2)  [unwired: 7 in]
    n103 = call <vilib>:"Set Duty Cycle.vi"("Duty Cycle"=w125, "PWM Ref In"=w127) -> ("error out"=w180:errorcluster, "PWM Ref Out"=w186:T2)  [unwired: 7 in]
    n104 = Merge Errors(w180, w181) -> (w179:errorcluster)
    n105 = xnode "PWM 2"("Duty Cycle"="Duty Cycle 2", "Frequency [Hz]"=w96) -> ()  [unwired: 1 in, 1 out]
    n106 = xnode "PWM"("Duty Cycle"="Duty Cycle", "Frequency [Hz]"=w96) -> ()  [unwired: 1 in, 1 out]
    n107 = xnode "Analog input (1 sample) 3"() -> ("stallBlanco (A/AI2 (Pin 7))"=w135:dbl, "stallRojo (A/AI3 (Pin 9))"=w134:dbl)  [unwired: 1 in, 1 out]
    "stallBlanco (A/AI2 (Pin 7))" <- w135
    "stallRojo (A/AI3 (Pin 9))" <- w134
    n108 = Bundle("Double"=w90, w99, "Counter Value"=w100, "seconds since 1Jan1904"=w189, "Double"=w89, w152, w151) -> (w156:T25)  [unwired: 1 in]
    n109 = shared-variable ".\\RT Variables.lvlib\\Stop RT Loops"() -> (w188:bool)  [unwired: 1 in, 1 out]
    n110 = xnode "Button"() -> ("Value"=w98:bool)  [unwired: 1 in, 1 out]
    n111 = shared-variable ".\\RT Variables.lvlib\\Data"(w156, error in=w179) -> (error out=w187:errorcluster)
    n112 = Greater?(x=w134, y=100.0) -> (0:w131:bool)
    n113 = Greater?(x=w135, y=100.0) -> (0:w132:bool)
    n114 = Or(x=w187, y=w188) -> (x .or. y?=w176:bool)
    n115 = Or(x=w132, y=w131) -> (x .or. y?=w133:bool)
    n116 = Or(x=w98, y=w133) -> (x .or. y?=w130:bool)
    n117 = Or(x=w176, y=w130) -> (x .or. y?=w175:bool)
  }
  n118 = while {
    shift-right: [w598] -> w54
    shift-left: w13 -> [w596]
    tunnel: [w597] -> w55
    tunnel: w2 -> [w595]
    shift-right: [w594] -> _
    shift-left: enum16{"Connect", "Send"}."Connect" ("Message states") -> [w599]
    stop <- w600 stop-if-true
    # "Data sending loop"
    n119 = case shown="\"Connect\"" w599 {
      tunnel: [w604 w619] -> w597
      tunnel: [w602 w617] -> w598
      tunnel: [w608 w620] -> w594
      tunnel: w596 -> [_ w626]
      tunnel: w595 -> [w605 w625]
      frame "Connect" {
        # "Attempts connection with the UI every 5 seconds, once successful, proceeds to Send state."
        n120 = Create Network Stream Writer Endpoint(5:5000 ("timeout in ms (-1)"), 7:4096 ("writer buffer size"), 8:w605, 9:T26 {"Double"=0.0, "dbl Scaled Value"=0.0, "Output"=0.0, "seconds since 1Jan1904"=timestamp(0 s since 1904-01-01), 0.0, 0.0, 0.0} ("Data"), 11:"data writer" ("writer name")) -> (0:w606:errorcluster, 3:w603:refnum<k21>)  [unwired: 2 in]
        n121 = case shown="Error" w606 {
          selector: w606 -> [w611 _]
          tunnel: [enum16{"Connect", "Send"}."Send" ("Message states") enum16{"Connect", "Send"}."Connect" ("Message states")] -> w608
          tunnel: [w611 errorcluster {"status"=FALSE, "code"=0, "source"=""} ("error IO")] -> w604
          tunnel: w603 -> [w613 _]
          tunnel: [w613 w614] -> w602
          frame No Error {
          }
          frame Error {
            w614 = refnum<k21> refnum  # writer endpoint
          }
        }
      }
      frame "Send" {
        # "Sends deterministic loop acquired data to the UI."
        n122 = shared-variable ".\\RT Variables.lvlib\\Data"(error in=w625) -> (w622:T26, error out=w624:errorcluster)
        n123 = Unbundle By Name(w624) -> ("code"=w623:i32)
        n124 = case shown="0, Default" w623 {
          tunnel: [w639 w641] -> w621
          tunnel: [w638 w640] -> w618
          tunnel: w626 -> [w637 w640]
          tunnel: w624 -> [w636 w641]
          tunnel: w622 -> [w635 _]
          frame 0, Default {
            n125 = shared-variable-write(w637, w636, w635) -> (w638:refnum<k21>, w639:errorcluster)  [unwired: 1 in, 1 out]
          }
          frame -2220 {
            n126 = Wait (ms)(milliseconds to wait=u32 10) -> ()  [unwired: 1 out]
          }
        }
        n127 = case shown="Error" w621 {
          selector: w621 -> [w629 w633]
          tunnel: [enum16{"Connect", "Send"}."Send" ("Message states") enum16{"Connect", "Send"}."Connect" ("Message states")] -> w620
          tunnel: [w629 errorcluster {"status"=FALSE, "code"=0, "source"=""} ("error IO")] -> w619
          tunnel: w618 -> [w627 w632]
          tunnel: [w627 w630] -> w617
          frame No Error {
          }
          frame Error {
            w630 = refnum<k21> refnum  # writer endpoint
            n128 = Destroy Stream Endpoint(8:w633, 11:w632) -> ()  [unwired: 1 out]
          }
        }
      }
    }
    n129 = shared-variable ".\\RT Variables.lvlib\\Stop RT Loops"() -> (w600:bool)  [unwired: 1 in, 1 out]
  }
  n130 = while {
    tunnel: [w645] -> w51
    shift-right: [w650] -> _
    shift-left: refnum<k21> refnum ("reader endpoint") -> [w648]
    shift-right: [w649] -> _
    shift-left: enum16{"Connect", "Receive"}."Connect" ("Message states") -> [w651]
    tunnel: w2 -> [w647]
    tunnel: w2 -> [w643]
    stop <- w644 stop-if-true
    # "Message loop"
    n131 = case shown="\"Receive\"" w651 {
      tunnel: [w658 w683] -> w646
      tunnel: [w656 w684] -> w650
      tunnel: [w665 w680] -> w649
      tunnel: w648 -> [_ w679]
      tunnel: w647 -> [_ w682]
      tunnel: [FALSE ("Stop RT Loops") w681] -> w644
      tunnel: w643 -> [_ w676]
      frame "Connect" {
        # "Attempts connection with the UI every 5 seconds, once successful, proceeds to Receive state."
        n132 = Bundle("", variant, variant) -> (w661:cluster{string, variant, variant})  [unwired: 1 in]
        n133 = Create Network Stream Reader Endpoint(5:5000 ("timeout in ms (-1)"), 7:4096 ("reader buffer size"), 9:w661, 11:"message reader" ("reader name")) -> (0:w660:errorcluster, 3:w655:refnum<k21>)  [unwired: 3 in]
        n134 = case shown="Error" w660 {
          selector: w660 -> [w670 _]
          tunnel: [enum16{"Connect", "Receive"}."Receive" ("Message states") enum16{"Connect", "Receive"}."Connect" ("Message states")] -> w665
          tunnel: [w669 errorcluster {"status"=FALSE, "code"=0, "source"=""} ("error IO")] -> w658
          tunnel: [w668 refnum<k21> refnum ("reader endpoint")] -> w656
          tunnel: w655 -> [w668 _]
          frame No Error {
            n135 = shared-variable ".\\RT Variables.lvlib\\2setpoint"(w668, error in=w670) -> (error out=w669:errorcluster)
          }
          frame Error {
          }
        }
      }
      frame "Receive" {
        # "Receives messages from the UI."
        n136 = shared-variable-read(w679, w682) -> (w678:refnum<k21>, w685:errorcluster, w675:cluster{string, variant, variant})  [unwired: 1 in, 1 out]
        n137 = Unbundle(w675) -> (w687:string, w686:variant, w677:variant)
        n138 = case shown="\"Vector Setpoints\"" w687 {
          tunnel: w686 -> [_ w708 w723 w729 w747]
          tunnel: w685 -> [w691 w710 w712 w728 w741]
          tunnel: [w690 w705 w719 w730 w737] -> w683
          tunnel: [refnum<k21> refnum ("reader endpoint") refnum<k21> refnum ("reader endpoint") w718 w736 w745] -> w684
          tunnel: w678 -> [w689 w704 w718 w736 w745]
          tunnel: [FALSE ("Stop RT Loops") w707 FALSE ("Stop RT Loops") FALSE ("Stop RT Loops") FALSE ("Stop RT Loops")] -> w681
          tunnel: [enum16{"Connect", "Receive"}."Connect" ("Message states") enum16{"Connect", "Receive"}."Receive" ("Message states") enum16{"Connect", "Receive"}."Receive" ("Message states") enum16{"Connect", "Receive"}."Receive" ("Message states") enum16{"Connect", "Receive"}."Receive" ("Message states")] -> w680
          tunnel: w677 -> [_ w700 w711 w732 w740]
          tunnel: w676 -> [_ w699 _ _ _]
          frame "Disconnect UI", Default {
            n139 = Destroy Stream Endpoint(8:w691, 11:w689) -> (0:w690:errorcluster)
          }
          frame "Stop" {
            n140 = Variant To Data(error in=w699, type=TRUE ("Stop RT Loops"), Variant=w700) -> (data=w697:bool, error out=w701:errorcluster)
            n141 = Variant To Data(error in=w710, type=TRUE ("Stop RT Loops"), Variant=w708) -> (data=w707:bool, error out=w709:errorcluster)
            n142 = shared-variable ".\\RT Variables.lvlib\\Stop RT Loops"(w707, error in=w709) -> (error out=w695:errorcluster)
            n143 = shared-variable ".\\RT Variables.lvlib\\Stop RT Loops"(w697, error in=w701) -> (error out=w696:errorcluster)
            n144 = Merge Errors(w695, w696) -> (w694:errorcluster)
            n145 = Destroy Stream Endpoint(8:w694, 11:w704) -> (0:w705:errorcluster)
          }
          frame "Update setpoint" {
            n146 = Variant To Data(error in=w712, type=0.0, Variant=w723) -> (data=w721:dbl, error out=w720:errorcluster)
            n147 = Variant To Data(error in=w712, type=0.0, Variant=w711) -> (data=w714:dbl, error out=w713:errorcluster)
            n148 = shared-variable ".\\RT Variables.lvlib\\Setpoint"(w721, error in=w720) -> (error out=w719:errorcluster)
            n149 = shared-variable ".\\RT Variables.lvlib\\Setpoint2"(w714, error in=w713) -> ()  [unwired: 1 out]
          }
          frame "Vector Setpoints" {
            n150 = Variant To Data(error in=w728, type=dbl[][][] [], Variant=w729) -> (data=w726:dbl[][][])  [unwired: 1 out]
            "vectores" <- w726
            n151 = Variant To Data(error in=w728, type=0.0, Variant=w732) -> (data=w731:dbl)  [unwired: 1 out]
            n152 = Index Array(array=w726) -> (element #1=w725:dbl[][], element #2=w724:dbl[][])  [unwired: 6 in]
            "subarray" <- w725
            "subarray 2" <- w724
            n153 = shared-variable ".\\RT Variables.lvlib\\Tiempo"(w731) -> (error out=w730:errorcluster)  [unwired: 1 in]
            n154 = shared-variable "myRIO-1900\\Untitled Library 7.lvlib\\subarray 2"(w724) -> ()  [unwired: 1 in, 1 out]
            n155 = shared-variable "myRIO-1900\\Untitled Library 6.lvlib\\subarray"(w725) -> ()  [unwired: 1 in, 1 out]
          }
          frame "Homing" {
            n156 = Variant To Data(error in=w741, type=TRUE, Variant=w747) -> (data=w739:bool, error out=w738:errorcluster)
            n157 = Variant To Data(error in=w741, type=0.0, Variant=w740) -> ()  [unwired: 2 out]
            n158 = shared-variable ".\\RT Variables.lvlib\\Homing"(w739, error in=w738) -> (error out=w737:errorcluster)
          }
        }
      }
    }
    n159 = case shown="No Error" w646 {
      selector: w646 -> [w652 w653]
      tunnel: [w652 w653] -> w645
      frame No Error {
        # "No action required."
      }
      frame Error {
        # "Stops RT in case of error."
        n160 = shared-variable ".\\RT Variables.lvlib\\Stop RT Loops"(TRUE ("Stop RT Loops")) -> ()  [unwired: 1 in, 1 out]
      }
    }
  }
  n161 = Destroy Stream Endpoint(8:w55, 11:w54) -> (0:w52:errorcluster)
  n162 = node-c288(w58) -> ()  [unwired: 1 out]
  n163 = case shown="Error" w47 {
    selector: w47 -> [w748 w749]
    tunnel: [w748 w749] -> w9
    frame No Error {
      # "No action required."
    }
    frame Error {
      # "Destroys Message network stream to stop Message loop, in case of error."
      n164 = shared-variable ".\\RT Variables.lvlib\\2setpoint"() -> (w750:refnum<k21>)  [unwired: 1 in, 1 out]
      n165 = Destroy Stream Endpoint(11:w750) -> ()  [unwired: 1 in, 1 out]
    }
  }
  n166 = call <vilib>:"Stop.vi"("error in (no error)"=w9, "Encoder Ref In"=w39) -> ("error out"=w40:errorcluster, "Encoder Ref Out"=w41:T9)  [unwired: 8 in]
  n167 = call <vilib>:"Stop.vi"("error in (no error)"=w9, "Encoder Ref In"=w8) -> ("error out"=w11:errorcluster, "Encoder Ref Out"=w12:T9)  [unwired: 8 in]
  n168 = call <vilib>:"Close.vi"("error in (no error)"=w40, "Encoder Ref In"=w41) -> ("error out"=w34:errorcluster)  [unwired: 9 in]
  n169 = call <vilib>:"Close.vi"("error in (no error)"=w11, "Encoder Ref In"=w12) -> ("error out"=w10:errorcluster)  [unwired: 9 in]
  n170 = call <vilib>:"Close.vi"("error in (no error)"=w34, "PWM Ref In"=w31) -> ("error out"=w33:errorcluster)  [unwired: 9 in]
  n171 = call <vilib>:"Close.vi"("error in (no error)"=w10, "PWM Ref In"=w7) -> ("error out"=w6:errorcluster)  [unwired: 9 in]
  n172 = Merge Errors(w52, w51, w33, w6) -> (w50:errorcluster)
  n173 = shared-variable "myRIO-1900\\Network Shared Variables.lvlib\\error IO"(w50) -> ()  [unwired: 1 in, 1 out]
